vi "findEdge.vi"(0 "reference":refnum<class "Graph.lvclass">, 1 "point2D":T1 {"y" format="%.2f"; "x" format="%.2f"}, 2 "GraphicsRef":refnum<class "Graphics.lvclass">, 5 "error in (no error)":errorcluster) -> (14 "reference out":refnum<class "Graph.lvclass">, 15 "edge":refnum<class "AbstractEdge.lvclass">, 16 "found":bool, 19 "error out":errorcluster)   [LabVIEW 2012, in "Graph.lvclass"]
doc: "Finds an edge containing the given point.\n @param p a point\n @return an edge containing p or null if no edges contain p\n */\n public Edge findEdge(Point2D p)"
uses:
  <resource>/Framework/Providers/Open_GDS/UML/Graph_class/Graph.lvclass
  <resource>/Framework/Providers/Open_GDS/UML/General/Point/Point Point2D.ctl
  <resource>/Framework/Providers/Open_GDS/UML/AbstractEdge_class/AbstractEdge.lvclass
  <resource>/Framework/Providers/Open_GDS/UML/Graphics_class/Graphics.lvclass
  <resource>/Framework/Providers/Open_GDS/UML/GeneralPathEdge_class/GeneralPathEdge.lvclass
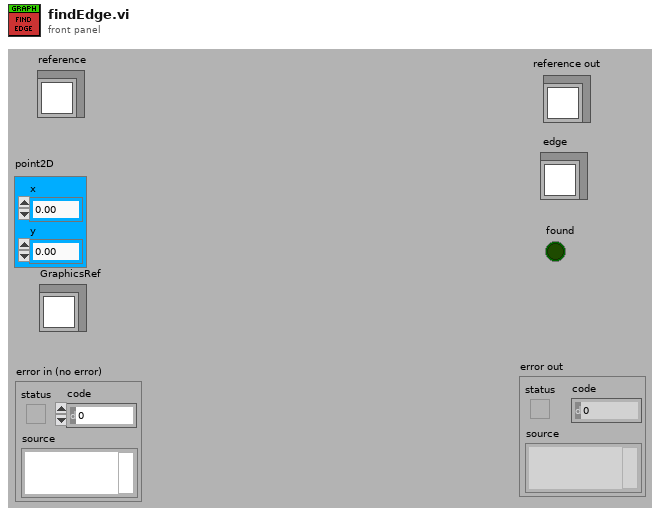
[diagram p1: front panel]
types:
  T1 = typedef "Point Point2D.ctl" = cluster{"x":dbl, "y":dbl}
  T2 = typedef "Graph.lvclass/ObjectAttributes.ctl" = cluster{"nodes":refnum<class "AbstractNode.lvclass">[], "edges":refnum<class "AbstractEdge.lvclass">[], "nodesToBeRemoved":refnum<class "AbstractNode.lvclass">[], "edgesToBeRemoved":refnum<class "AbstractEdge.lvclass">[], "needsLayout":bool, "LayoutNodes":refnum<class "AbstractNode.lvclass">[]}
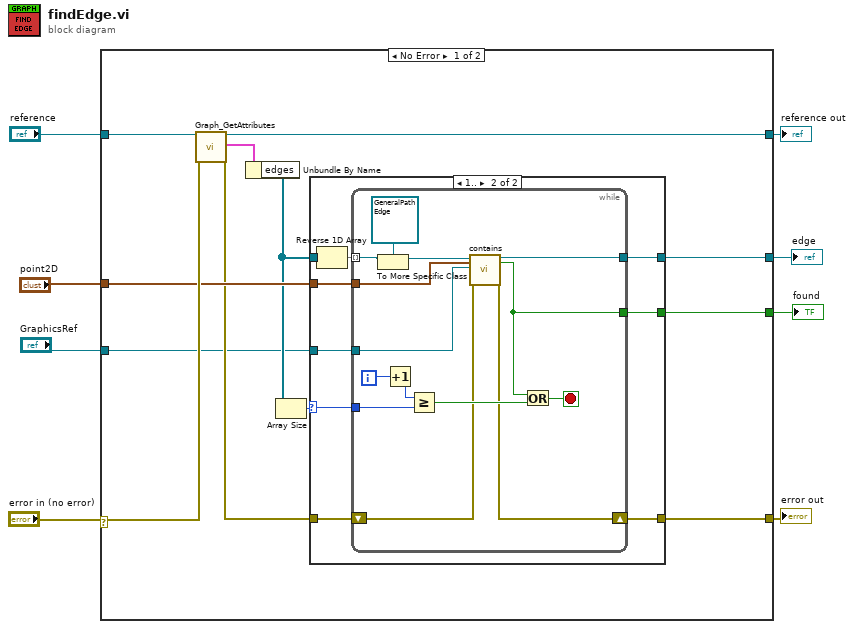
[diagram p0: block diagram]
diagram:
  n1 = case shown="No Error" "error in (no error)" {
    selector: "error in (no error)" -> [w17 w45]
    tunnel: "reference" -> [w20 w46]
    tunnel: [w19 w45] -> w7
    tunnel: [w18 w46] -> w6
    tunnel: "point2D" -> [w16 _]
    tunnel: [w15 _] -> w3
    tunnel: [w14 _] -> w2
    tunnel: "GraphicsRef" -> [w9 _]
    frame No Error {
      n2 = call <resource>:"Graph_GetAttributes.vi"("reference in"=w20, "error in (no error)"=w17) -> ("reference out"=w18:refnum<class "Graph.lvclass">, "Attributes"=w13:T2, "error out"=w11:errorcluster)  [unwired: 15 out]
      n3 = Unbundle By Name(w13) -> ("edges"=w12:refnum<class "AbstractEdge.lvclass">[])
      n4 = Array Size(array=w12) -> (size(s)=w10:i32)
      n5 = case shown="1.." w10 {
        selector: w10 -> [_ w23]
        tunnel: w12 -> [_ w30]
        tunnel: w11 -> [w21 w29]
        tunnel: [w21 w28] -> w19
        tunnel: [_ w27] -> w15
        tunnel: w16 -> [_ w26]
        tunnel: [_ w25] -> w14
        tunnel: w9 -> [_ w22]
        frame 0, Default {
        }
        frame 1.. {
          n6 = Reverse 1D Array(array=w30) -> (reversed array=w24:refnum<class "AbstractEdge.lvclass">[])
          n7 = while {
            tunnel: w23 -> [w42]
            tunnel: w24 -> [w32] mode=indexing
            shift-right: [w38] -> w28
            shift-left: w29 -> [w39]
            tunnel: [w37] -> w27
            tunnel: w26 -> [w36]
            tunnel: [w35] -> w25
            tunnel: w22 -> [w31]
            i -> [w44]
            stop <- w40 stop-if-true
            n8 = To More Specific Class(target class=refnum<class "GeneralPathEdge.lvclass"> refnum ("reference out"), reference=w32) -> (specific class reference=w34:refnum<class "GeneralPathEdge.lvclass">)  [unwired: 1 in, 1 out]
            n9 = Increment(x=w44) -> (x+1=w43:i32)
            n10 = Greater Or Equal?(x=w43, y=w42) -> (x >= y?=w41:bool)
            n11 = call-dynamic "contains.vi"("reference"=w34, "point2D"=w36, "GraphicsRef"=w31, "error in (no error)"=w39) -> ("reference out"=w37:refnum<class "GeneralPathEdge.lvclass">, "contains"=w35:bool, "error out"=w38:errorcluster)  [unwired: 13 in]
            n12 = Or(x=w35, y=w41) -> (x .or. y?=w40:bool)
          }
        }
      }
    }
    frame Error {
    }
  }
  "reference out" <- w6
  "error out" <- w7
  "found" <- w2
  "edge" <- w3
